vi "LTE Configure Standard.vi"(0 "RFmx Handle In":refnum<k21>, 1 "Selector String":string, 5 "LTE Standard Configuration":T1={"Link Direction"=1, "Duplex Scheme"=0, "Uplink Downlink Configuration"=0, "Band"=1, "PUSCH Auto Resource Block Detection Enabled"=1, "Auto DMRS Detection Enabled"=0, "Downlink Auto Cell ID Detection Enabled"=0, "Component Carrier Configurations"=[{"Bandwidth (Hz)"=10000000.0, "Cell ID"=0, "PUSCH Modulation Type"=0, "PUSCH Resource Block Offset"=0, "PUSCH Number of Resource Blocks"=-1, "Downlink Test Model"=0}]} {"Downlink Auto Cell ID Detection Enabled" items=["False", "True"]; "Link Direction" items=["Downlink", "Uplink"]; "Auto DMRS Detection Enabled" items=["False", "True"]; "PUSCH Auto Resource Block Detection Enabled" items=["False", "True"]; "Component Carrier Configurations"."Downlink Test Model" items=["TM1.1", "TM1.2", "TM2", "TM 2a", "TM 3.1", "TM 3.2", "TM 3.3", "TM 3.1a"]; "Component Carrier Configurations"."PUSCH Modulation Type" items=["QPSK", "16 QAM", "64 QAM", "256 QAM", "1024 QAM"]; "Component Carrier Configurations"."Bandwidth (Hz)" items=["200.0 k"=200000.0, "1.4 M"=1400000.0, "3.0 M"=3000000.0, "5.0 M"=5000000.0, "10.0 M"=10000000.0, "15.0 M"=15000000.0, "20.0 M"=20000000.0]; "Uplink Downlink Configuration" items=["0", "1", "2", "3", "4", "5", "6"]; "Duplex Scheme" items=["FDD", "TDD", "LAA"]}, 11 "error in (no error)":errorcluster) -> (4 "RFmx Handle Out":refnum<k21>, 15 "error out":errorcluster)   [LabVIEW 2016, in "RFmxLTE.lvlib"]
uses:
  RFmxLTE.lvlib
  Typedefs/LTE Standard Configuration.ctl
  Typedefs/LTE Component Carrier Configuration.ctl
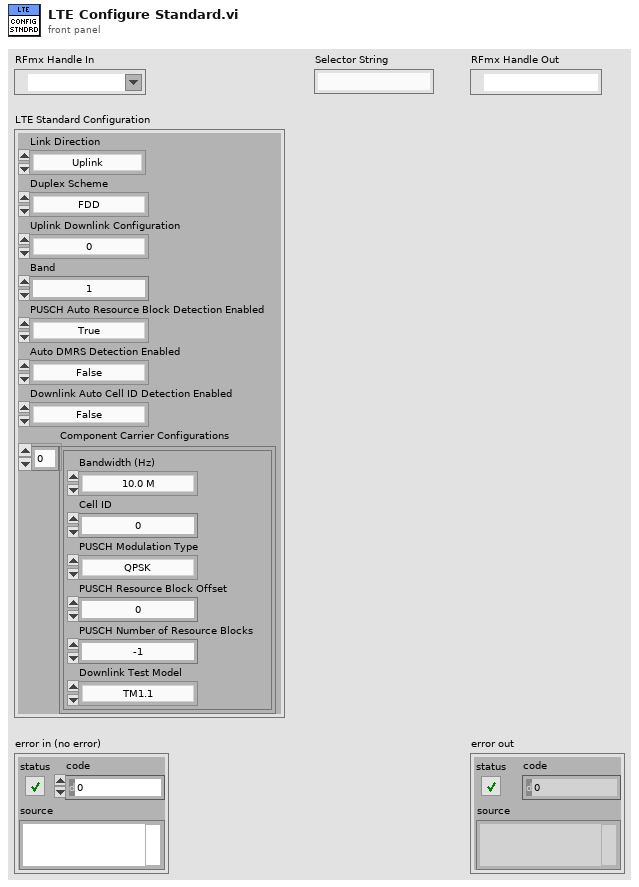
[diagram p1: front panel]
types:
  T1 = typedef "RFmxLTE.lvlib/LTE Standard Configuration.ctl" = cluster{"Link Direction":i32, "Duplex Scheme":i32, "Uplink Downlink Configuration":i32, "Band":i32, "PUSCH Auto Resource Block Detection Enabled":i32, "Auto DMRS Detection Enabled":i32, "Downlink Auto Cell ID Detection Enabled":i32, "Component Carrier Configurations":T2[]}
  T2 = typedef "RFmxLTE.lvlib/LTE Component Carrier Configuration.ctl" = cluster{"Bandwidth (Hz)":dbl, "Cell ID":i32, "PUSCH Modulation Type":i32, "PUSCH Resource Block Offset":i32, "PUSCH Number of Resource Blocks":i32, "Downlink Test Model":i32}
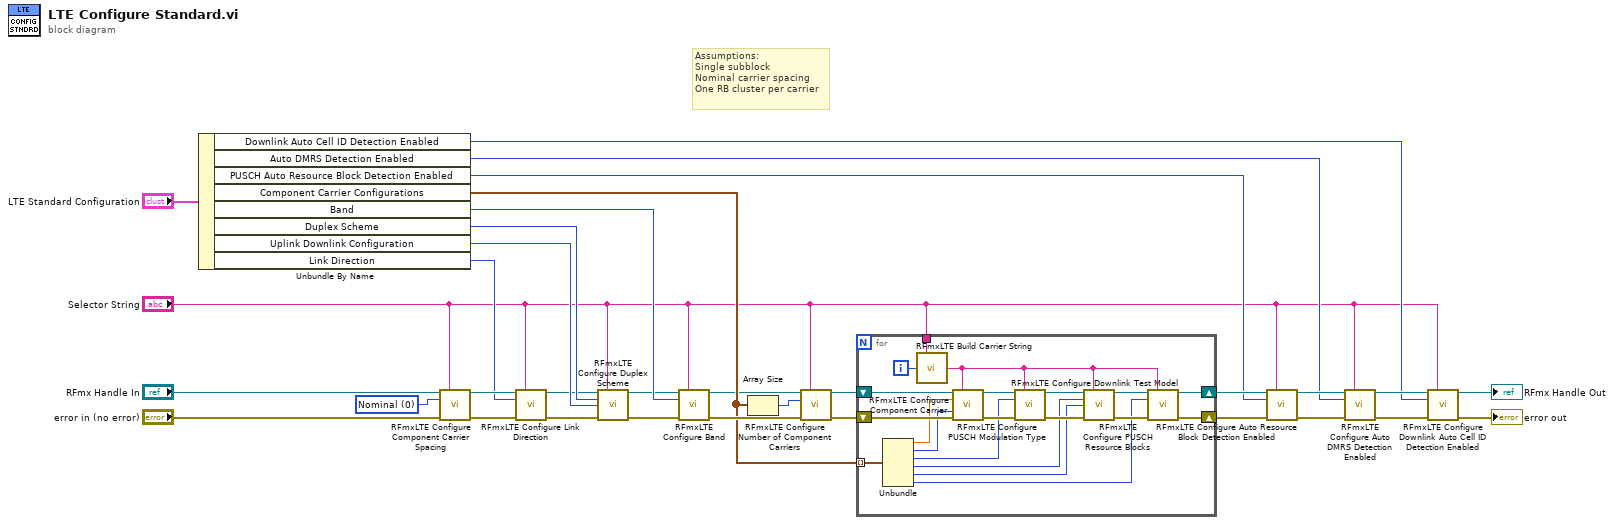
[diagram p0: block diagram]
diagram:
  w18 = 0 items=["Nominal", "Minimum", "User"] ("Component Carrier Spacing Type")
  # "Assumptions:\nSingle subblock\nNominal carrier spacing\nOne RB cluster per carrier"
  n1 = Unbundle By Name("LTE Standard Configuration") -> ("Downlink Auto Cell ID Detection Enabled"=w2:i32, "Auto DMRS Detection Enabled"=w10:i32, "PUSCH Auto Resource Block Detection Enabled"=w11:i32, "Component Carrier Configurations"=w14:T2[], "Band"=w19:i32, "Duplex Scheme"=w21:i32, "Uplink Downlink Configuration"=w20:i32, "Link Direction"=w5:i32)
  n2 = call <vilib>:"RFmxLTE Configure Component Carrier Spacing.vi"("Instrument Handle In"="RFmx Handle In", "Selector String"="Selector String", "Component Carrier Spacing Type"=w18, "error in (no error)"="error in (no error)") -> ("Instrument Handle Out"=w6:refnum<k21>, "error out"=w25:errorcluster)  [unwired: 10 in]
  n3 = call <vilib>:"RFmxLTE Configure Link Direction.vi"("Instrument Handle In"=w6, "Selector String"="Selector String", "Link Direction"=w5, "error in (no error)"=w25) -> ("Instrument Handle Out"=w7:refnum<k21>, "error out"=w26:errorcluster)  [unwired: 10 in]
  n4 = call <vilib>:"RFmxLTE Configure Duplex Scheme.vi"("Instrument Handle In"=w7, "Selector String"="Selector String", "Duplex Scheme"=w21, "Uplink Downlink Configuration"=w20, "error in (no error)"=w26) -> ("Instrument Handle Out"=w16:refnum<k21>, "error out"=w32:errorcluster)  [unwired: 9 in]
  n5 = call <vilib>:"RFmxLTE Configure Band.vi"("Instrument Handle In"=w16, "Selector String"="Selector String", "Band"=w19, "error in (no error)"=w32) -> ("Instrument Handle Out"=w9:refnum<k21>, "error out"=w28:errorcluster)  [unwired: 10 in]
  n6 = Array Size(array=w14) -> (size(s)=w17:i32)
  n7 = call <vilib>:"RFmxLTE Configure Number of Component Carriers.vi"("Instrument Handle In"=w9, "Selector String"="Selector String", "Number of Component Carriers"=w17, "error in (no error)"=w28) -> ("Instrument Handle Out"=w15:refnum<k21>, "error out"=w31:errorcluster)  [unwired: 10 in]
  n8 = for {
    shift-right: [w48] -> w30
    shift-left: w31 -> [w52]
    tunnel: w14 -> [w45] mode=indexing
    shift-right: [w34] -> w13
    shift-left: w15 -> [w46]
    tunnel: "Selector String" -> [w37]
    i -> [w47]
    n9 = Unbundle(w45) -> ("Bandwidth (Hz)"=w44:dbl, "Cell ID"=w43:i32, "PUSCH Modulation Type"=w41:i32, "PUSCH Resource Block Offset"=w39:i32, "PUSCH Number of Resource Blocks"=w38:i32, "Downlink Test Model"=w33:i32)
    n10 = call <vilib>:"RFmxLTE Build Carrier String.vi"("Selector String"=w37, "Carrier Number"=w47) -> ("Selector String Out"=w35:string)  [unwired: 13 in]
    n11 = call <vilib>:"RFmxLTE Configure Component Carrier.vi"("Instrument Handle In"=w46, "Selector String"=w35, "Component Carrier Bandwidth (Hz)"=w44, "Cell ID"=w43, "error in (no error)"=w52) -> ("Instrument Handle Out"=w42:refnum<k21>, "error out"=w51:errorcluster)  [unwired: 9 in]
    n12 = call <vilib>:"RFmxLTE Configure PUSCH Modulation Type.vi"("Instrument Handle In"=w42, "Selector String"=w35, "Modulation Type"=w41, "error in (no error)"=w51) -> ("Instrument Handle Out"=w40:refnum<k21>, "error out"=w50:errorcluster)  [unwired: 10 in]
    n13 = call <vilib>:"RFmxLTE Configure PUSCH Resource Blocks.vi"("Instrument Handle In"=w40, "Selector String"=w35, "Resource Block Offset"=w39, "Number of Resource Blocks"=w38, "error in (no error)"=w50) -> ("Instrument Handle Out"=w36:refnum<k21>, "error out"=w49:errorcluster)  [unwired: 9 in]
    n14 = call <vilib>:"RFmxLTE Configure Downlink Test Model.vi"("Instrument Handle In"=w36, "Selector String"=w35, "DL Test Model"=w33, "error in (no error)"=w49) -> ("Instrument Handle Out"=w34:refnum<k21>, "error out"=w48:errorcluster)  [unwired: 10 in]
  }
  n15 = call <vilib>:"RFmxLTE Configure Auto Resource Block Detection Enabled.vi"("Instrument Handle In"=w13, "Selector String"="Selector String", "Auto Resource Block Detection Enabled"=w11, "error in (no error)"=w30) -> ("Instrument Handle Out"=w12:refnum<k21>, "error out"=w29:errorcluster)  [unwired: 10 in]
  n16 = call <vilib>:"RFmxLTE Configure Auto DMRS Detection Enabled.vi"("Instrument Handle In"=w12, "Selector String"="Selector String", "Auto DMRS Detection Enabled"=w10, "error in (no error)"=w29) -> ("Instrument Handle Out"=w4:refnum<k21>, "error out"=w24:errorcluster)  [unwired: 10 in]
  n17 = call <vilib>:"RFmxLTE Configure Downlink Auto Cell ID Detection Enabled.vi"("Instrument Handle In"=w4, "Selector String"="Selector String", "Auto Cell ID Detection Enabled"=w2, "error in (no error)"=w24) -> ("Instrument Handle Out"=→"RFmx Handle Out":refnum<k21>, "error out"=→"error out":errorcluster)  [unwired: 10 in]
